vi "Verify as JSON.vi"(5 "Label":string, 7 "Options":refnum<class "Options.lvclass">, 8 "error in":errorcluster, 10 "Anything":variant, 11 "LUnit Test Case In":refnum<class "Test Case.lvclass">) -> (0 "error out":errorcluster, 3 "LUnit Test Case Out":refnum<class "Test Case.lvclass">)   [LabVIEW 2020, in "LUnit.Extension.lvlib"]
doc: "Takes in anything. Flattens it to JSON."
uses:
  LUnit.Extension.lvlib
  <vilib>/Astemes/LUnit/Test Case.lvclass
  Approval Tests/Options/Options.lvclass
  Approval Tests/Options/Options.lvclass/Options.ctl
  Approval Tests/Naming Data/Naming Data.lvclass/Naming Data.ctl
  <vilib>/Astemes/LUnit/Test Case.lvclass/Test Case.ctl
  Approval Tests/Approval Tests.lvlib
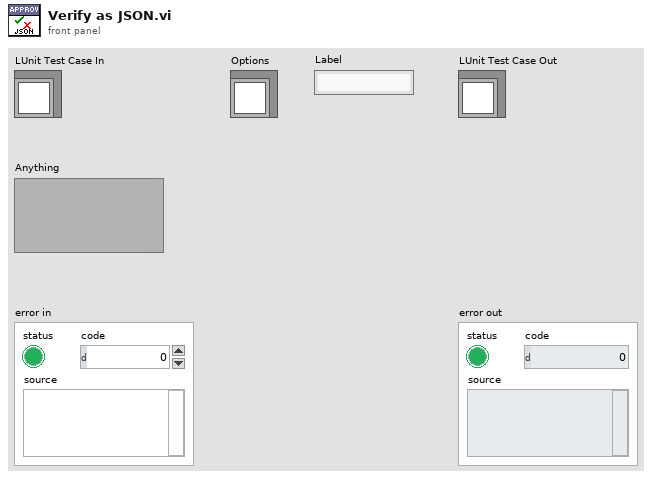
[diagram p1: front panel]
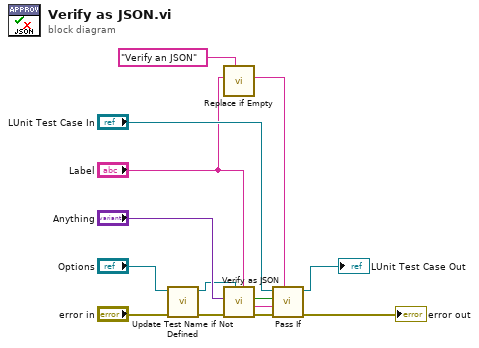
[diagram p0: block diagram]
diagram:
  n1 = call "Update Test Name if Not Defined.vi"("error in"="error in", "Options in"="Options") -> ("error out"=w11:errorcluster, "Options out"=w4:refnum<class "Options.lvclass">)  [unwired: 8 in]
  n2 = call "Replace if Empty.vi"("if empty"="Verify an JSON", "Text in"="Label") -> ("Text out"=w1:string)  [unwired: 9 in]
  n3 = call "Verify as JSON.vi"("Label"="Label", "Approval Tests.lvlib:Options.lvclass"=w4, "error in"=w11, "Anything"="Anything") -> ("error out"=w12:errorcluster, "Failure Message"=w7:string, "Passed?"=w8:bool)  [unwired: 5 in]
  n4 = call <vilib>:"Pass If.vi"("Description"=w1, "error in (no error)"=w12, "Message"=w7, "Pass?"=w8, "LUnit Test Case In"="LUnit Test Case In") -> ("error out"=→"error out":errorcluster, "LUnit Test Case Out"=→"LUnit Test Case Out":refnum<class "Test Case.lvclass">)  [unwired: 5 in]
